vi "Create Outline.vi"(5 "Drawable":refnum<vi>, 7 "3D Pie Property":T4, 8 "error in (no error)":errorcluster, 10 "Plot Representation In":T1, 11 "Plot Object In":refnum<vi>) -> (0 "error out":errorcluster, 2 "Plot Representation Out":T1, 3 "Plot Object Out":refnum<vi>, 4 "Outline Object Out":refnum<vi>)   [LabVIEW 2020, in "3D Pie.lvclass"]
uses:
  <vilib>/Math Plots/3D Math Plots/3D Pie/3D Pie/3D Pie.lvclass
  <vilib>/Math Plots/3D Math Plots/3D Pie/3D Pie/Typedef/3D Pie Property.ctl
  <vilib>/Math Plots/3D Math Plots/3D Plot/3D Plot/Typedef/Line Type.ctl
  <vilib>/Math Plots/3D Math Plots/3D Plot/3D Plot/Typedef/Plot Representation.ctl
  <vilib>/Math Plots/3D Math Plots/3D Plot/3D Plot/Typedef/Range Clusters.ctl
  <vilib>/Math Plots/3D Math Plots/3D Plot/3D Plot/Typedef/Mesh Data.ctl
  <vilib>/picture/3D Picture Control/NI_3D Picture Control.lvlib
  <vilib>/Math Plots/3D Math Plots/3D Plot/3D Plot/3D Plot.lvclass
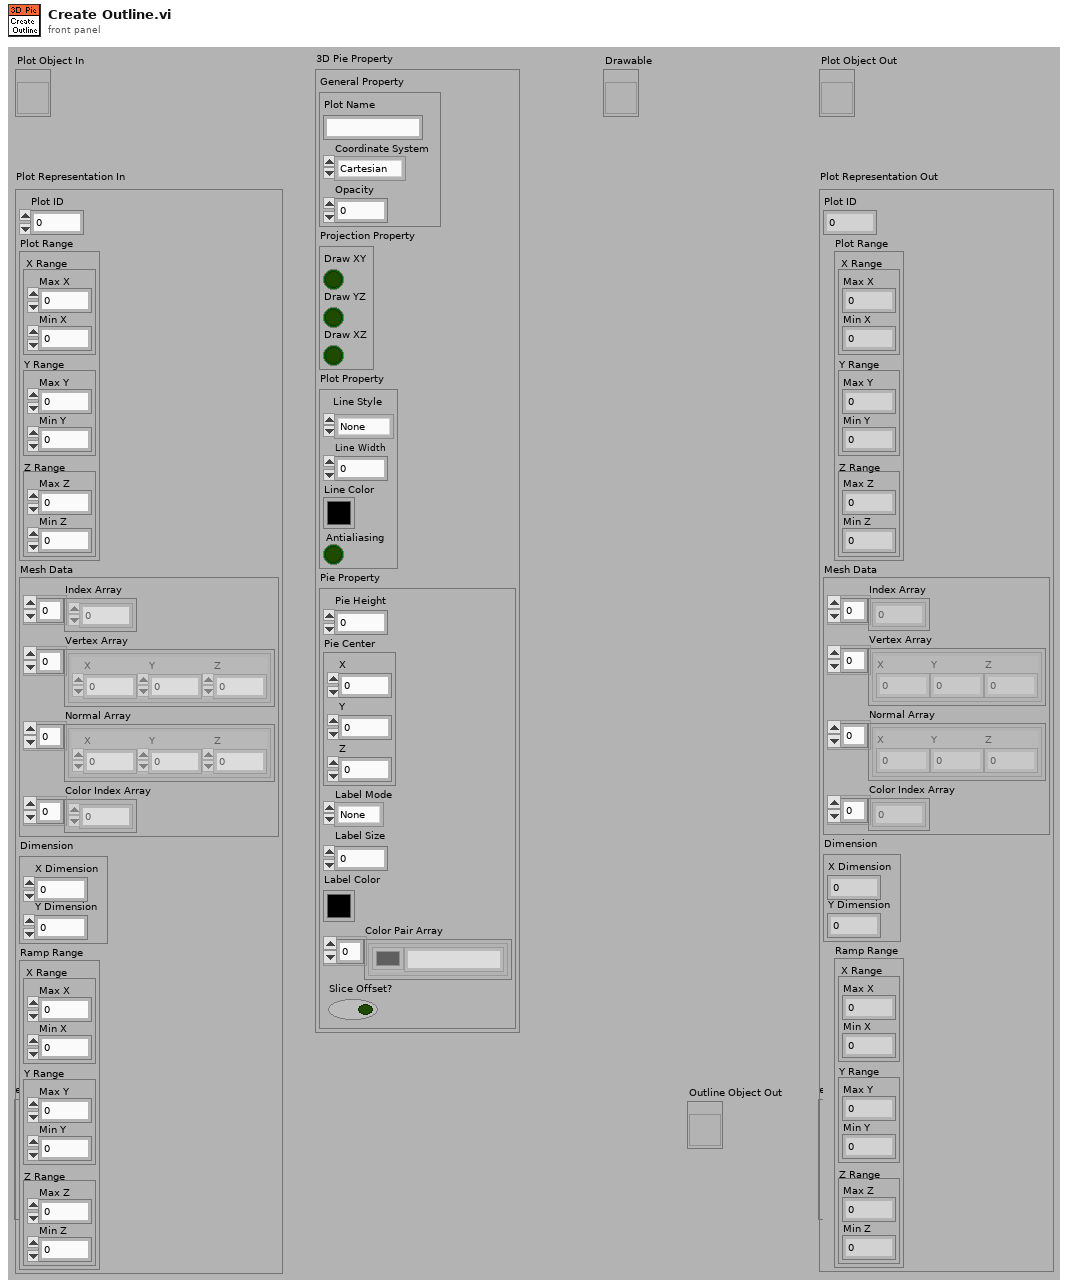
[diagram p1: front panel]
types:
  T1 = typedef "3D Plot.lvclass/Plot Representation.ctl" = cluster{"Plot ID":i32, "Plot Range":T2, "Mesh Data":T3, "Dimension":cluster{"X Dimension":i32, "Y Dimension":i32}, "Ramp Range":T2}
  T2 = typedef "3D Plot.lvclass/Range Clusters.ctl" = cluster{"X Range":cluster{"Max X":sgl, "Min X":sgl}, "Y Range":cluster{"Max Y":sgl, "Min Y":sgl}, "Z Range":cluster{"Max Z":sgl, "Min Z":sgl}}
  T3 = typedef "3D Plot.lvclass/Mesh Data.ctl" = cluster{"Index Array":u32[], "Vertex Array":cluster{"X":sgl, "Y":sgl, "Z":sgl}[], "Normal Array":cluster{"X":sgl, "Y":sgl, "Z":sgl}[], "Color Index Array":i32[]}
  T4 = typedef "3D Pie.lvclass/3D Pie Property.ctl" = cluster{"General Property":cluster{"Plot Name":string, "Coordinate System":enum16{"Cartesian", "Cylindrical", "Spherical"}, "Opacity":sgl}, "Projection Property":cluster{"Draw XY":bool, "Draw YZ":bool, "Draw XZ":bool}, "Plot Property":cluster{"Line Style":T5, "Line Width":sgl, "Line Color":u32, "Antialiasing":bool}, "Pie Property":cluster{"Pie Height":sgl, "Pie Center":cluster{"X":sgl, "Y":sgl, "Z":sgl}, "Label Mode":enum16{"None", "Show Percentage", "Show String"}, "Label Size":u16, "Label Color":u32, "Color Pair Array":cluster{"Color":u32, "String":string}[], "Slice Offset?":bool}}
  T5 = typedef "3D Plot.lvclass/Line Type.ctl" = enum16{"None", "Solid", "Dash", "Dot", "Dash Dot"}
  T6 = enum16{"Points", "Lines", "Line Strip", "Line Loop", "Triangles", "Triangle Strip", "Triangle Fan", "Quads", "Quad Strip", "Polygon"}
  T7 = enum16{"Overall", "Per Primitive", "Per Vertex", "Binding Off"}
  T8 = typedef "LV3DPointTypeDef.ctl" = cluster{"X":sgl, "Y":sgl, "Z":sgl}
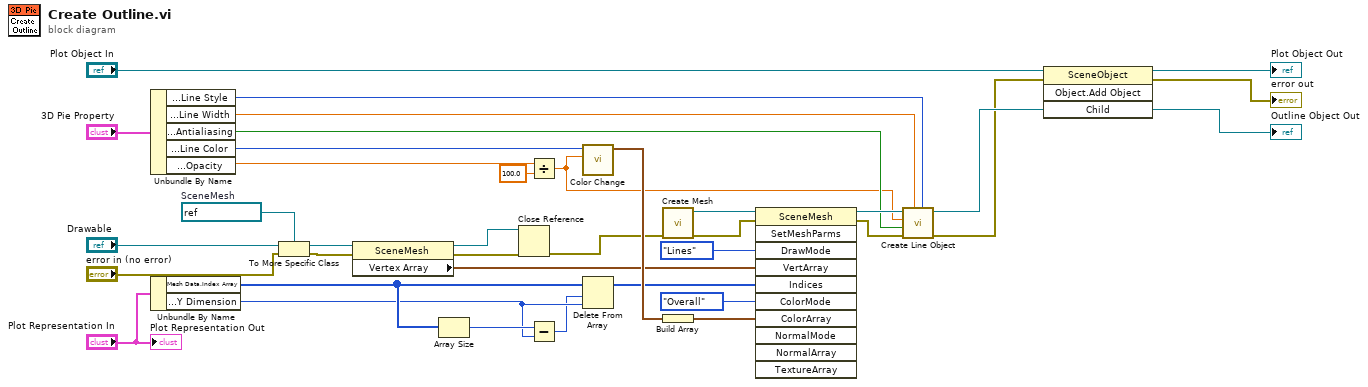
[diagram p0: block diagram]
diagram:
  w8 = refnum<vi> refnum  # SceneMesh
  n1 = Unbundle By Name("3D Pie Property") -> ("Plot Property.Line Style"=w18:T5, "Plot Property.Line Width"=w19:sgl, "Plot Property.Antialiasing"=w16:bool, "Plot Property.Line Color"=w29:u32, "General Property.Opacity"=w17:sgl)
  n2 = Unbundle By Name("Plot Representation In") -> ("Mesh Data.Index Array"=w14:u32[], "Dimension.Y Dimension"=w12:i32)
  n3 = To More Specific Class(target class=w8, reference="Drawable", error in="error in (no error)") -> (specific class reference=w7:refnum<vi>, error out=w3:errorcluster)
  n4 = property class="SceneMesh"(reference=w7, error in=w3) -> (reference out=w6:refnum<vi>, error out=w2:errorcluster, "Vertex Array"=w5:T8[])
  n5 = Array Size(array=w14) -> (size(s)=w13:i32)
  n6 = Close Reference(reference=w6, error in (no error)=w2) -> (error out=w1:errorcluster)
  n7 = Divide(x=w17, y=sgl 100.0) -> (x/y=w15:sgl)
  n8 = Subtract(x=w13, y=w12) -> (x-y=w11:i32)
  n9 = call <vilib>:"Color Change.vi"("Alpha"=w15, "Color"=w29) -> ("RGBA"=w28:cluster{"R":sgl, "G":sgl, "B":sgl, "A":sgl})  [unwired: 9 out]
  n10 = Delete From Array(array=w14, length=w11, index=w12) -> (array with subset deleted=w10:u32[])  [unwired: 1 out]
  n11 = call <vilib>:"Create Mesh.vi"("error in (no error)"=w1) -> ("error out"=w36:errorcluster, "New Mesh Refnum"=w37:refnum<vi>)  [unwired: 9 out]
  n12 = Build Array(w28) -> (w27:cluster{"R":sgl, "G":sgl, "B":sgl, "A":sgl}[])
  n13 = invoke class="SceneMesh" method="SetMeshParms"(reference=w37, error in=w36, "DrawMode"=T6."Lines" ("Draw Mode"), "VertArray"=w5, "Indices"=w10, "ColorMode"=T7."Overall" ("Color Binding Mode"), "ColorArray"=w27) -> (reference out=w23:refnum<vi>, error out=w24:errorcluster)  [unwired: 4 in, 9 out]
  n14 = call <vilib>:"Create Line Object.vi"("Line Style"=w18, "Line Width"=w19, "error in (no error)"=w24, "Antialiasing"=w16, "Alpha"=w15, "Mesh Ref In"=w23) -> ("error out"=w21:errorcluster, "Object Ref Out"=w22:refnum<vi>)  [unwired: 4 out]
  n15 = invoke class="SceneObject" method="Object.Add Object"(reference="Plot Object In", error in=w21, "Child"=w22) -> (reference out=→"Plot Object Out":refnum<vi>, error out=→"error out":errorcluster, "Child"=→"Outline Object Out":refnum<vi>)  [unwired: 1 in, 1 out]
  "Plot Representation Out" <- "Plot Representation In"
